vi "dfd_HEADER_H.vi"() -> ()   [LabVIEW 2017, in "NI_DigFilterTemp.lvlib"]
uses:
  <vilib>/addons/Digital Filter Design/NI_DigFilterTemp.lvlib
panel:
  in  "String":string="/* ==================================================================== \n * Title:     %FilterBlkName%.h                                                  \n *                                                                      \n * Purpose:                                                             \n *            Present typedefs, global variables declaration and       \n * function prototypes.                                                 \n *                                                                      \n * Copyright 2008 National Instruments Corporation. All rights reserved.       \n * ==================================================================== \n */\n\n#ifndef __%FilterBlkName%_%FilterType%_H__\n#define __%FilterBlkName%_%FilterType%_H__\n\n#include <stdio.h>\n#include <math.h>\n#include <stdlib.h>\n\n#include \"nidfdtyp.h\"\n\n#ifdef __cplusplus\nextern \"C\"{\n#endif\n\n/* ----Typedef---- */\ntypedef %StateType%* %FilterBlkName%_State;\n\n/* ----Create/Dispose State---- */\n%FilterBlkName%_State %FilterBlkName%_CreateState ( );\nvoid %FilterBlkName%_DisposeState (%FilterBlkName%_State state);\n\n/* ----Initialize State---- */\nvoid %FilterBlkName%_InitState (%FilterBlkName%_State state);\n\n/* ----Filter Implementation---- */\n%OutType% %FilterBlkName%_Filtering (%InType% sampleIn, %FilterBlkName%_State state);\n\n/* ----Demo Program---- */\n/* void main()\n * {\n *     //Declare and create State\n *     %FilterBlkName%_State state;\n *     state = %FilterBlkName%_CreateState();\n *\n *     ...\n *\n *     //Initialize State\n *     %FilterBlkName%_InitState (state);\n *\n *     ...\n *\n *     //Processing\n *     while ()\n *     {\n *         ...\n *         y = %FilterBlkName%_Filtering(x, state);\n *         ...\n *     };\n *\n *     ...\n *\n *     //Dispose State\n *     %FilterBlkName%_DisposeState (state);\n *\n *     ...\n *\n *     return;\n * }\n */\n\n#ifdef __cplusplus\n}\n#endif\n\n#endif //#ifndef __%FilterBlkName%_%FilterType%_H__\n"
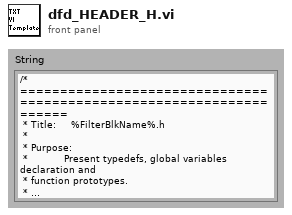
[diagram p1: front panel]
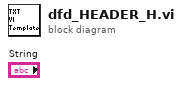
[diagram p0: block diagram]
diagram:
